vi "Coffee_machine.vi"(0 "1 Cup":bool, 1 "Water Level":dbl(slide) scale=0.0..100.0, 2 "Milk Level":dbl(slide) scale=0.0..100.0, 5 "1 Carafe":bool, 7 "Type":u32(knob) scale=0.0..2.0, 9 "Power":bool, 11 "Error In":errorcluster, 12 "Bean Level":dbl(slide) scale=0.0..100.0) -> (3 "Heating":bool, 4 "Low Water":bool, 6 "Low Bean":bool, 8 "Low Milk":bool, 10 "Purging":bool, 15 "Error Out":errorcluster)   [LabVIEW 2020]
uses:
  Typedef's/Q_Operations.ctl
  Typedef's/Data Cluster.ctl
  <vilib>/Utility/config.llb/Write Key (Boolean).vi
  <vilib>/Utility/config.llb/Read Key (Double).vi
  <vilib>/Utility/config.llb/Read Key (Boolean).vi
  <vilib>/Utility/config.llb/NI_LVConfig.lvlib
panel:
  in  "Power Shutdown?":bool
  out "Dispensing":bool
  out "Brewing":bool
  out "Grinding":bool
  out "Total Cups":dbl
  out "Elapsed Time":dbl format="%#.0f"
  out "Dispenser":dbl(slide) scale=0.0..60.0
  in  "Chamber":dbl(slide) scale=0.0..60.0
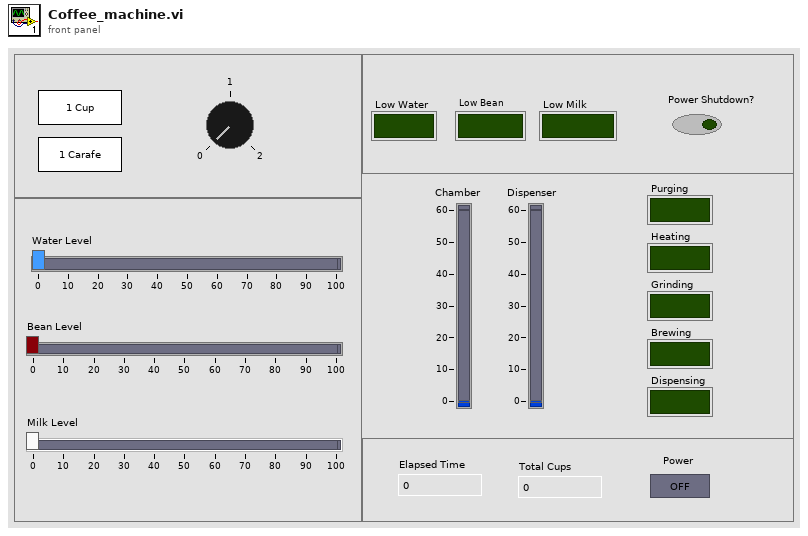
[diagram p1: front panel]
types:
  T1 = typedef "Data Cluster.ctl" = cluster{"Bean Level":dbl, "Chamber":dbl, "Dispenser":dbl, "Milk Level":dbl, "Elapsed Time":dbl, "Total Cups":dbl, "Water Level":dbl, "1 Carafe":bool, "1 Cup":bool, "Low Bean":bool, "Low Water":bool, "Low Milk":bool, "Power Shutdown?":bool, "Heating":bool, "Grinding":bool, "Brewing":bool, "Dispensing":bool, "Purging":bool, "Power":bool, "Type":u32, "Timer":cluster{"Previous Time":dbl, "Elapsed Time":dbl, "Start":bool, "Pause":bool, "Set Time":dbl}, "Sequecne":string[], "Value":dbl}
  T2 = typedef "Q_Operations.ctl" = enum16{"Create Q", "Enqueue", "Dequeue", "Enqueue N ele", "Enstack N ele", "Flush Q", "Destroy Q"}
  T3 = enum8{"Enabled", "Disabled", "Disabled and Grayed Out"}
  T4 = typedef "NI_LVConfig.lvlib/Config Data RefNum.ctl" = refnum<k1>
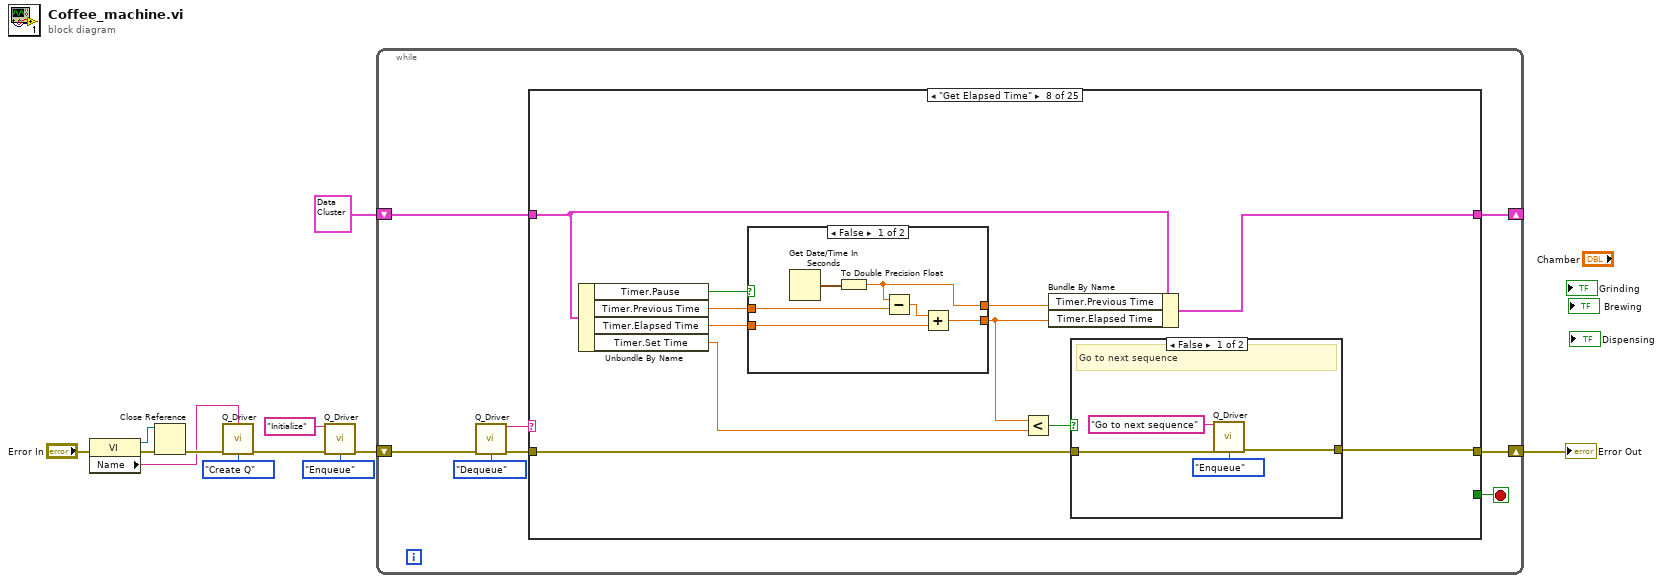
[diagram p0: block diagram]
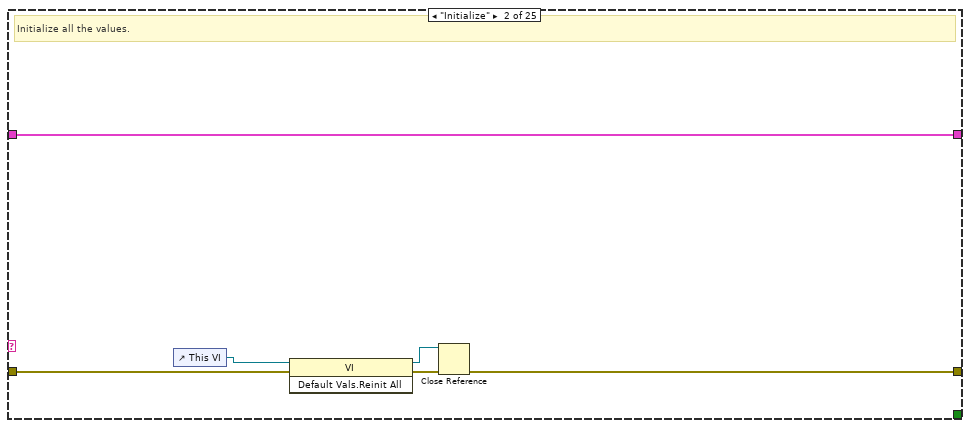
[diagram p3: hidden frame]
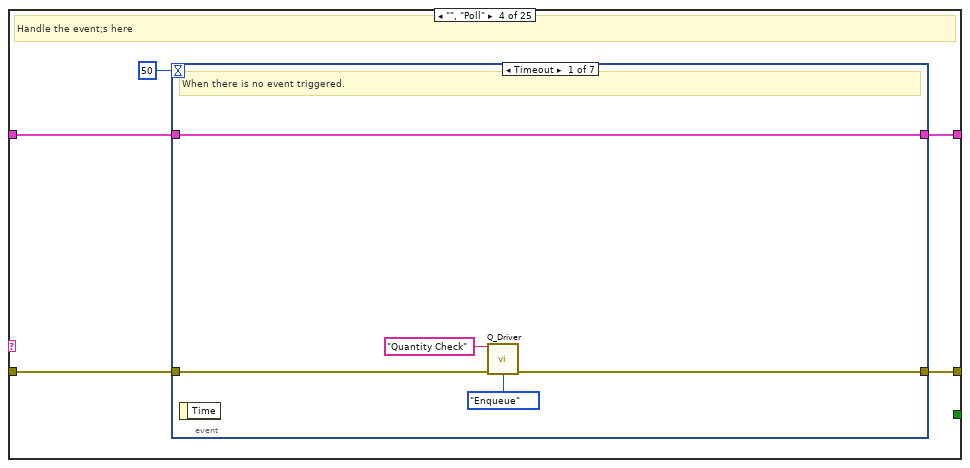
[diagram p5: hidden frame]
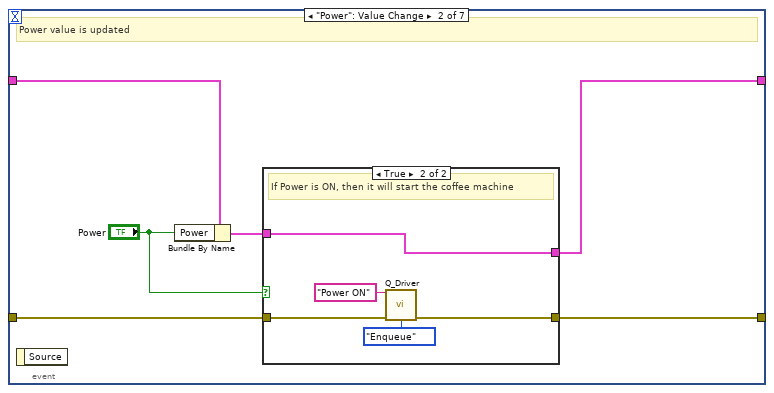
[diagram p6: hidden frame]
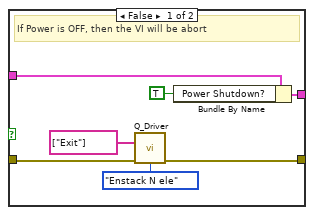
[diagram p7: hidden frame]
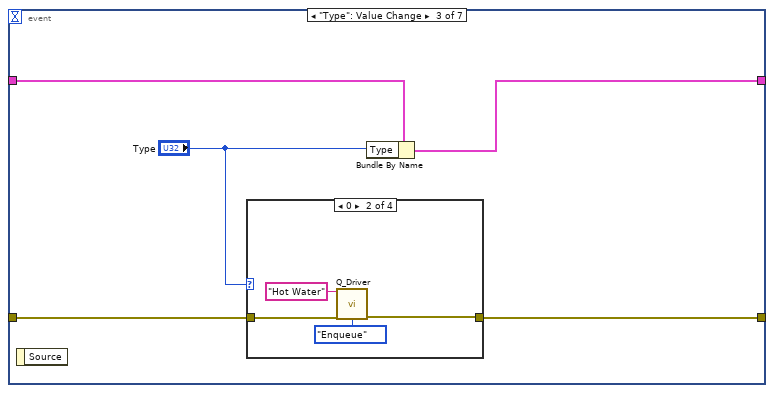
[diagram p8: hidden frame]
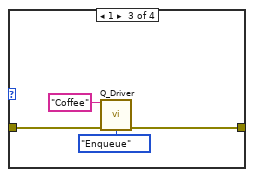
[diagram p10: hidden frame]
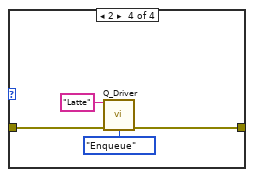
[diagram p11: hidden frame]
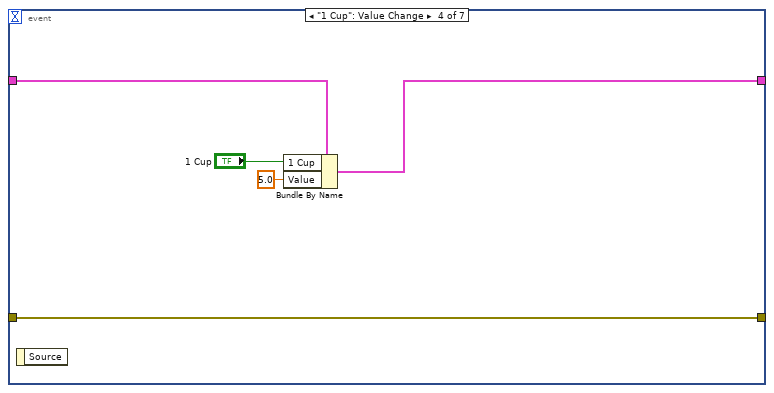
[diagram p12: hidden frame]
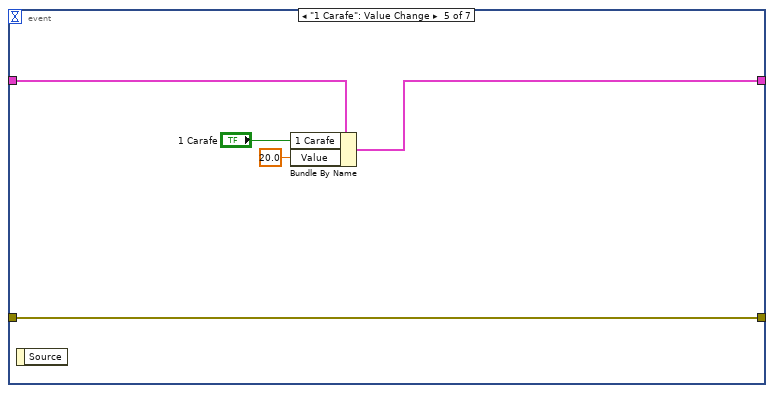
[diagram p13: hidden frame]
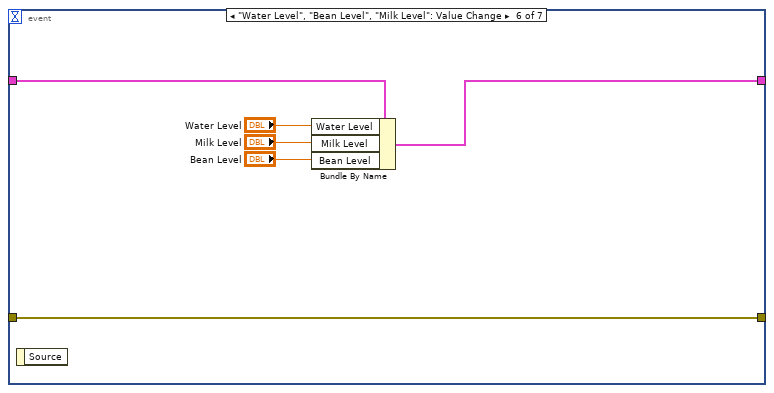
[diagram p14: hidden frame]
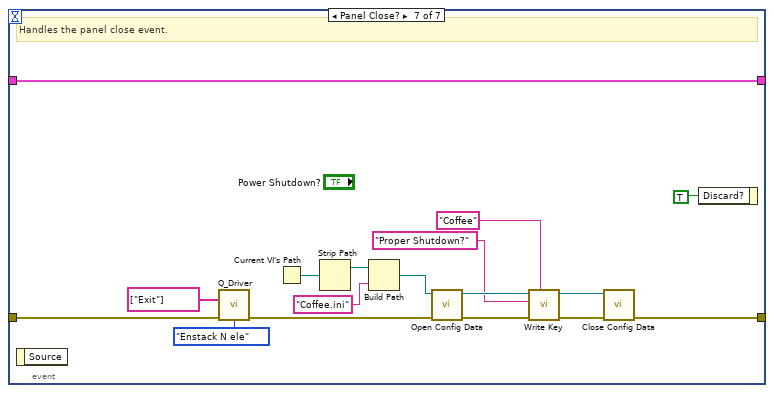
[diagram p15: hidden frame]
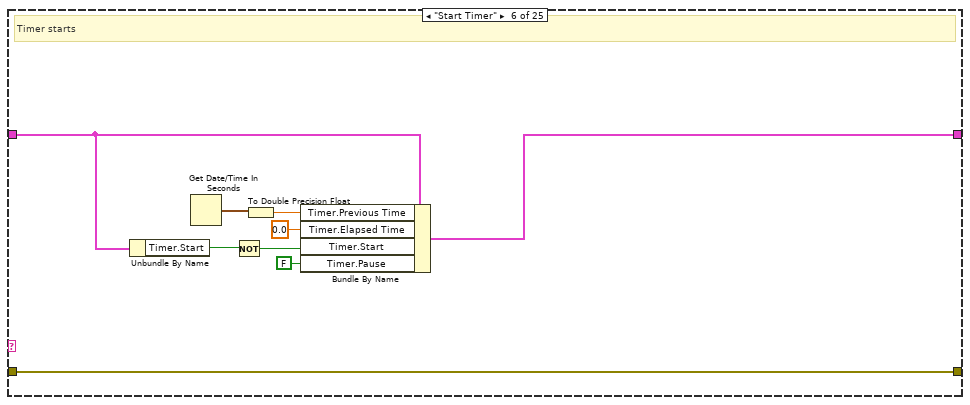
[diagram p17: hidden frame]
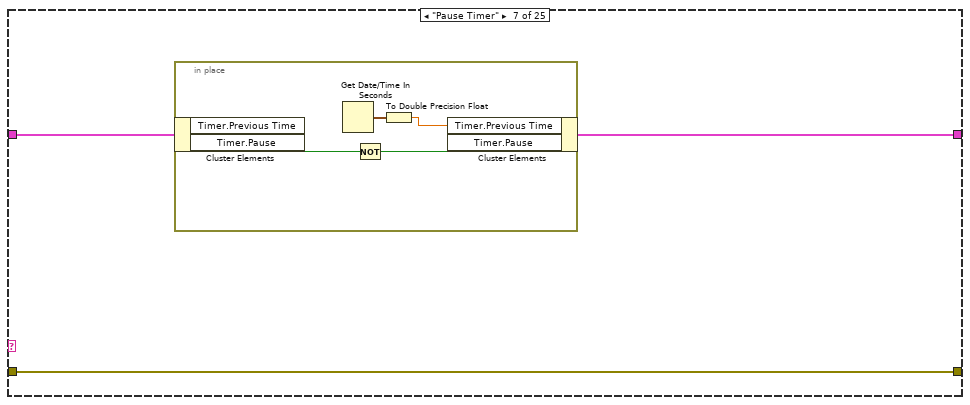
[diagram p18: hidden frame]
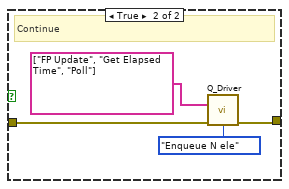
[diagram p19: hidden frame]
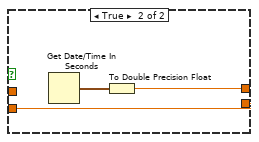
[diagram p20: hidden frame]
diagram:
  n1 = property class="VI"(error in="Error In") -> (reference out=w9:refnum<vi>, error out=w11:errorcluster, "Name"=w6:string)  [unwired: 1 in]
  n2 = Close Reference(reference=w9, error in (no error)=w11) -> (error out=w10:errorcluster)
  n3 = call "Q_Driver.vi"("Name"=w6, "Error In"=w10, "Operations"=Q_Operations."Create Q") -> ("Error Out"=w8:errorcluster)  [unwired: 11 in, 1 out]
  n4 = call "Q_Driver.vi"("State"="Initialize", "Error In"=w8, "Operations"=Q_Operations."Enqueue") -> ("Error Out"=w5:errorcluster)  [unwired: 11 in, 1 out]
  n5 = while {
    shift-right: [w16] -> w2
    shift-left: w5 -> [w19]
    shift-right: [w13] -> _
    shift-left: T1 {"Bean Level"=0.0, "Chamber"=0.0, "Dispenser"=0.0, "Milk Level"=0.0, "Elapsed Time"=0.0, "Total Cups"=0.0, "Water Level"=0.0, "1 Carafe"=FALSE, "1 Cup"=FALSE, "Low Bean"=FALSE, "Low Water"=FALSE, "Low Milk"=FALSE, "Power Shutdown?"=FALSE, "Heating"=FALSE, "Grinding"=FALSE, "Brewing"=FALSE, "Dispensing"=FALSE, "Purging"=FALSE, "Power"=FALSE, "Type"=0, "Timer"={"Previous Time"=0.0, "Elapsed Time"=0.0, "Start"=FALSE, "Pause"=FALSE, "Set Time"=0.0}, "Sequecne"=[], "Value"=0.0} -> [w14]
    stop <- w15 stop-if-true
    n6 = call "Q_Driver.vi"("Error In"=w19, "Operations"=Q_Operations."Dequeue") -> ("Dequeued Element"=w17:string, "Error Out"=w20:errorcluster)  [unwired: 12 in]
    n7 = case shown="\"Get Elapsed Time\"" w17 {
      tunnel: w20 -> [w22 w27 w30 w34 w111 w120 w123 w129 w157 w172 w181 w208 w216 w230 w241 w248 w271 w287 w289 w296 w298 w301 w307 w309 w311]
      tunnel: [w22 w23 w30 w33 w111 w120 w123 w128 w157 w164 w178 w209 w217 w237 w238 w247 w266 w287 w289 w296 w298 w302 w307 w309 w311] -> w16
      tunnel: [_ _ _ _ _ _ _ _ _ _ _ _ _ _ _ _ _ _ _ _ _ TRUE _ _ _] -> w15
      tunnel: w14 -> [w21 w24 w29 w32 w110 w118 w122 w134 w156 w165 w177 w211 w222 w233 w245 w256 w284 w286 w288 w295 w297 w304 w306 w308 w310]
      tunnel: [w21 w24 w29 w31 w110 w119 w121 w135 w156 w166 w176 w212 w223 w234 w245 w256 w285 w286 w288 w295 w297 w304 w306 w308 w310] -> w13
      frame "/**** Initialize ****/" {
      }
      frame "Initialize" {
        # "Initialize all the values."
        n8 = control-ref of="This VI"() -> (w28:refnum<vi>)
        n9 = invoke class="VI" method="Default Vals.Reinit All"(reference=w28, error in=w27) -> (reference out=w25:refnum<vi>, error out=w26:errorcluster)  [unwired: 1 in, 1 out]
        n10 = Close Reference(reference=w25, error in (no error)=w26) -> (error out=w23:errorcluster)
      }
      frame "/****Events*****/" {
      }
      frame "", "Poll" {
        # "Handle the event;s here"
        n11 = event shown="[0] Timeout" {
          selector: _ -> [_ _ _ _ _ _ _]
          dyn-events: _ -> [_ _ _ _ _ _ _]
          timeout: 50 -> [_ _ _ _ _ _ _]
          tunnel: w34 -> [w36 w44 w60 w77 w82 w87 w109]
          tunnel: [w37 w45 w59 w77 w82 w87 w93] -> w33
          tunnel: w32 -> [w40 w46 w62 w78 w86 w91 w105]
          tunnel: [w40 w41 w63 w81 w84 w92 w105] -> w31
          event Timeout {
            # "When there is no event triggered."
            n12 = event-data() -> ()  [unwired: 1 in, 1 out]
            n13 = call "Q_Driver.vi"("State"="Quantity Check", "Error In"=w36, "Operations"=Q_Operations."Enqueue") -> ("Error Out"=w37:errorcluster)  [unwired: 11 in, 1 out]
          }
          event "Power": Value Change {
            # "Power value is updated"
            n14 = event-data() -> ()  [unwired: 1 in, 1 out]
            n15 = Bundle By Name(cluster=w46, "Power"="Power") -> (w42:T1)
            n16 = case shown="True" "Power" {
              tunnel: [w52 w58] -> w45
              tunnel: w44 -> [w53 w57]
              tunnel: w42 -> [w49 w54]
              tunnel: [w48 w54] -> w41
              frame False {
                # "If Power is OFF, then the VI will be abort"
                n17 = call "Q_Driver.vi"("States[]"=string[] ["Exit"], "Error In"=w53, "Operations"=Q_Operations."Enstack N ele") -> ("Error Out"=w52:errorcluster)  [unwired: 11 in, 1 out]
                n18 = Bundle By Name(cluster=w49, "Power Shutdown?"=TRUE) -> (w48:T1)
              }
              frame True {
                # "If Power is ON, then it will start the coffee machine"
                n19 = call "Q_Driver.vi"("State"="Power ON", "Error In"=w57, "Operations"=Q_Operations."Enqueue") -> ("Error Out"=w58:errorcluster)  [unwired: 11 in, 1 out]
              }
            }
          }
          event "Type": Value Change {
            n20 = event-data() -> ()  [unwired: 1 in, 1 out]
            n21 = case shown="0" "Type" {
              tunnel: w60 -> [w64 w68 w72 w76]
              tunnel: [w64 w67 w71 w75] -> w59
              frame Default {
              }
              frame 0 {
                n22 = call "Q_Driver.vi"("State"="Hot Water", "Error In"=w68, "Operations"=Q_Operations."Enqueue") -> ("Error Out"=w67:errorcluster)  [unwired: 11 in, 1 out]
              }
              frame 1 {
                n23 = call "Q_Driver.vi"("State"="Coffee", "Error In"=w72, "Operations"=Q_Operations."Enqueue") -> ("Error Out"=w71:errorcluster)  [unwired: 11 in, 1 out]
              }
              frame 2 {
                n24 = call "Q_Driver.vi"("State"="Latte", "Error In"=w76, "Operations"=Q_Operations."Enqueue") -> ("Error Out"=w75:errorcluster)  [unwired: 11 in, 1 out]
              }
            }
            n25 = Bundle By Name(cluster=w62, "Type"="Type") -> (w63:T1)
          }
          event "1 Cup": Value Change {
            n26 = event-data() -> ()  [unwired: 1 in, 1 out]
            n27 = Bundle By Name(cluster=w78, "1 Cup"="1 Cup", "Value"=5.0 ("Cup")) -> (w81:T1)
          }
          event "1 Carafe": Value Change {
            n28 = event-data() -> ()  [unwired: 1 in, 1 out]
            n29 = Bundle By Name(cluster=w86, "1 Carafe"="1 Carafe", "Value"=20.0) -> (w84:T1)
          }
          event "Water Level", "Bean Level", "Milk Level": Value Change {
            n30 = event-data() -> ()  [unwired: 1 in, 1 out]
            n31 = Bundle By Name(cluster=w91, "Water Level"="Water Level", "Milk Level"="Milk Level", "Bean Level"="Bean Level") -> (w92:T1)
          }
          event Panel Close? {
            # "Handles the panel close event."
            n32 = event-data() -> ()  [unwired: 1 in, 1 out]
            n33 = call "Q_Driver.vi"("States[]"=string[] ["Exit"], "Error In"=w109, "Operations"=Q_Operations."Enstack N ele") -> ("Error Out"=w100:errorcluster)  [unwired: 11 in, 1 out]
            n34 = Current VI's Path() -> (path=w102:path)
            n35 = Strip Path(path=w102) -> (stripped path=w103:path)  [unwired: 1 out]
            n36 = Build Path(base path=w103, name or relative path="Coffee.ini") -> (appended path=w104:path)
            n37 = call <vilib>:"Open Config Data.vi"("error in (no error)"=w100, "configuration file path"=w104) -> ("error out"=w99:errorcluster, "refnum"=w98:T4)  [unwired: 7 in, 1 out]
            n38 = call-poly <vilib>:"Write Key.vi"("section"="Coffee", "error in (no error)"=w99, "key"="Proper Shutdown?", "refnum"=w98) -> ("error out"=w94:errorcluster, "refnum out"=w95:T4)  [unwired: 5 in, 1 out]
            n39 = call <vilib>:"Close Config Data.vi"("error in (no error)"=w94, "refnum"=w95) -> ("error out"=w93:errorcluster)  [unwired: 8 in, 1 out]
            n40 = event-data("Discard?"=TRUE) -> ()  [unwired: 1 in, 1 out]
          }
        }
      }
      frame "/****Timer Operations*****/" {
      }
      frame "Start Timer" {
        # "Timer starts"
        n41 = Unbundle By Name(w118) -> ("Timer.Start"=w117:bool)
        n42 = Get Date/Time In Seconds() -> (seconds since 1Jan1904=w115:timestamp)
        n43 = Not(x=w117) -> (.not. x?=w116:bool)
        n44 = To Double Precision Float(number=w115) -> (double precision float=w114:dbl)
        n45 = Bundle By Name(cluster=w118, "Timer.Previous Time"=w114, "Timer.Elapsed Time"=0.0, "Timer.Start"=w116, "Timer.Pause"=FALSE) -> (w119:T1)
      }
      frame "Pause Timer" {
        n46 = in-place {
          n47 = in-place-cluster #1(w122) -> ("Timer.Pause"=w127:bool)  [unwired: 1 out]
          n48 = Get Date/Time In Seconds() -> (seconds since 1Jan1904=w125:timestamp)
          n49 = Not(x=w127) -> (.not. x?=w126:bool)
          n50 = To Double Precision Float(number=w125) -> (double precision float=w124:dbl)
          n51 = in-place-cluster #1("Timer.Previous Time"=w124, "Timer.Pause"=w126) -> (w121:T1)
        }
      }
      frame "Get Elapsed Time" {
        n52 = Unbundle By Name(w134) -> ("Timer.Pause"=w138:bool, "Timer.Previous Time"=w136:dbl, "Timer.Elapsed Time"=w137:dbl, "Timer.Set Time"=w131:dbl)
        n53 = case shown="False" w138 {
          tunnel: [w147 w153] -> w133
          tunnel: w137 -> [w151 w155]
          tunnel: w136 -> [w148 _]
          tunnel: [w149 w155] -> w132
          frame False {
            n54 = Get Date/Time In Seconds() -> (seconds since 1Jan1904=w152:timestamp)
            n55 = To Double Precision Float(number=w152) -> (double precision float=w147:dbl)
            n56 = Subtract(x=w147, y=w148) -> (x-y=w150:dbl)
            n57 = Add(x=w150, y=w151) -> (x+y=w149:dbl)
          }
          frame True {
            n58 = Get Date/Time In Seconds() -> (seconds since 1Jan1904=w154:timestamp)
            n59 = To Double Precision Float(number=w154) -> (double precision float=w153:dbl)
          }
        }
        n60 = Less?(x=w132, y=w131) -> (x < y?=w130:bool)
        n61 = Bundle By Name(cluster=w134, "Timer.Previous Time"=w133, "Timer.Elapsed Time"=w132) -> (w135:T1)
        n62 = case shown="False" w130 {
          tunnel: w129 -> [w142 w145]
          tunnel: [w141 w146] -> w128
          frame False {
            # "Go to next sequence"
            n63 = call "Q_Driver.vi"("State"="Go to next sequence", "Error In"=w142, "Operations"=Q_Operations."Enqueue") -> ("Error Out"=w141:errorcluster)  [unwired: 11 in, 1 out]
          }
          frame True {
            # "Continue"
            n64 = call "Q_Driver.vi"("States[]"=string[] ["FP Update", "Get Elapsed Time", "Poll"], "Error In"=w145, "Operations"=Q_Operations."Enqueue N ele") -> ("Error Out"=w146:errorcluster)  [unwired: 11 in, 1 out]
          }
        }
      }
      frame "/****Functionality****/" {
      }
      frame "Power ON" {
        n65 = Current VI's Path() -> (path=w175:path)
        n66 = Strip Path(path=w175) -> (stripped path=w174:path)  [unwired: 1 out]
        n67 = Build Path(base path=w174, name or relative path="Coffee.ini") -> (appended path=w171:path)
        n68 = call <vilib>:"Open Config Data.vi"("error in (no error)"=w172, "configuration file path"=w171) -> ("error out"=w169:errorcluster, "refnum"=w170:T4)  [unwired: 7 in, 1 out]
        n69 = call-poly <vilib>:"Read Key.vi"("section"="Coffee", "error in (no error)"=w169, "key"="Total Cups", "refnum"=w170) -> ("error out"=w161:errorcluster, "value"=w162:dbl, "refnum out"=w159:T4)  [unwired: 4 in, 1 out]
        n70 = call <vilib>:"Close Config Data.vi"("error in (no error)"=w161, "refnum"=w159) -> ("error out"=w160:errorcluster)  [unwired: 8 in, 1 out]
        n71 = Bundle By Name(cluster=w165, "Total Cups"=w162) -> (w166:T1)
        n72 = call "Q_Driver.vi"("States[]"=string[] ["FP Update", "Power Update"], "Error In"=w160, "Operations"=Q_Operations."Enqueue N ele") -> ("Error Out"=w164:errorcluster)  [unwired: 11 in, 1 out]
      }
      frame "Power Update" {
        # "Power status sequence is updated"
        n73 = Current VI's Path() -> (path=w185:path)
        n74 = Strip Path(path=w185) -> (stripped path=w186:path)  [unwired: 1 out]
        n75 = Build Path(base path=w186, name or relative path="Coffee.ini") -> (appended path=w187:path)
        n76 = call <vilib>:"Open Config Data.vi"("error in (no error)"=w181, "configuration file path"=w187) -> ("error out"=w189:errorcluster, "refnum"=w188:T4)  [unwired: 7 in, 1 out]
        n77 = call-poly <vilib>:"Read Key.vi"("section"="Coffee", "error in (no error)"=w189, "key"="Proper Shutdown?", "refnum"=w188) -> ("error out"=w179:errorcluster, "value"=w180:bool)  [unwired: 4 in, 2 out]
        n78 = case shown="False" w180 {
          tunnel: w179 -> [w195 w201]
          tunnel: [w196 w200] -> w178
          tunnel: w177 -> [w192 w197]
          tunnel: [w191 w197] -> w176
          frame False {
            # "If the VI is aborted , then Purging process starts"
            n79 = call "Q_Driver.vi"("States[]"=string[] ["Start Timer", "Purging", ""], "Error In"=w195, "Operations"=Q_Operations."Enqueue N ele") -> ("Error Out"=w196:errorcluster)  [unwired: 11 in, 1 out]
            n80 = Bundle By Name(cluster=w192, "Sequecne"=string[] ["Purging", "Heating"]) -> (w191:T1)
          }
          frame True {
            # "If Power is OFF, then Heating process starts"
            n81 = call "Q_Driver.vi"("States[]"=string[] ["Start Timer", "Heating"], "Error In"=w201, "Operations"=Q_Operations."Enqueue N ele") -> ("Error Out"=w200:errorcluster)  [unwired: 11 in, 1 out]
          }
        }
      }
      frame "Heating" {
        n82 = call "Q_Driver.vi"("State"="Get Elapsed Time" ("States[]"), "Error In"=w208, "Operations"=Q_Operations."Enqueue") -> ("Error Out"=w209:errorcluster)  [unwired: 11 in, 1 out]
        n83 = Bundle By Name(cluster=w211, "Purging"=FALSE, "Heating"=TRUE, "Chamber"=0.0, "Dispenser"=0.0, "Timer.Set Time"=5.0) -> (w212:T1)
      }
      frame "Purging" {
        n84 = call "Q_Driver.vi"("State"="Get Elapsed Time", "Error In"=w216, "Operations"=Q_Operations."Enqueue") -> ("Error Out"=w217:errorcluster)  [unwired: 11 in, 1 out]
        n85 = Bundle By Name(cluster=w222, "Heating"=FALSE, "Purging"=TRUE, "Chamber"=0.0, "Dispenser"=0.0, "Timer.Set Time"=4.0) -> (w223:T1)
      }
      frame "Go to next sequence" {
        n86 = Unbundle By Name(w233) -> ("Sequecne"=w231:string[])
        n87 = Delete From Array(array=w231, index=0) -> (array with subset deleted=w229:string[])  [unwired: 1 in, 1 out]
        n88 = Index Array(array=w229, index=0) -> (element=w225:string)
        n89 = Empty String/Path?(string/path=w225) -> (empty?=w227:bool)
        n90 = Select(t="Default state", s=w227, f=w225) -> (s? t:f=w224:string)
        n91 = Bundle By Name(cluster=w233, "Sequecne"=w229, "Timer.Elapsed Time"=0.0) -> (w234:T1)
        n92 = call "Q_Driver.vi"("State"=w224, "Error In"=w230, "Operations"=Q_Operations."Enqueue") -> ("Error Out"=w237:errorcluster)  [unwired: 11 in, 1 out]
      }
      frame "Default state" {
        n93 = control-ref of="This VI"() -> (w242:refnum<vi>)
        n94 = invoke class="VI" method="Default Vals.Reinit All"(reference=w242, error in=w241) -> (reference out=w244:refnum<vi>, error out=w243:errorcluster)  [unwired: 1 in, 1 out]
        n95 = Close Reference(reference=w244, error in (no error)=w243) -> (error out=w239:errorcluster)
        n96 = property on="Power" class="Bool (strict)"(error in=w239, "Value"=TRUE ("Power")) -> (error out=w238:errorcluster)  [unwired: 1 in, 1 out]
      }
      frame "Quantity Check" {
        w252 = 30.0 ("y")
        n97 = Unbundle By Name(w256) -> ("Water Level"=w255:dbl, "Bean Level"=w254:dbl, "Milk Level"=w253:dbl)
        n98 = Greater?(x=w255, y=w252) -> (0:w246:bool)
        n99 = Greater?(x=w254, y=w252) -> (0:w251:bool)
        n100 = Greater?(x=w253, y=w252) -> (0:w250:bool)
        n101 = Compound Arithmetic op=OR(w246, w251, w250) -> (w249:bool)
        n102 = case shown="False" w249 {
          tunnel: w248 -> [w258 w260]
          tunnel: [w257 w261] -> w247
          frame False {
            n103 = property on="Type" class="Knob (strict)"(error in=w258, "DisabledEnum"=T3."Disabled and Grayed Out" ("Disabled")) -> (error out=w257:errorcluster)  [unwired: 1 in, 1 out]
          }
          frame True {
            n104 = property on="Type" class="Knob (strict)"(error in=w260, "DisabledEnum"=T3."Enabled" ("Disabled")) -> (error out=w261:errorcluster)  [unwired: 1 in, 1 out]
          }
        }
      }
      frame "Hot Water" {
        n105 = Unbundle By Name(w284) -> ("Dispenser"=w283:dbl, "Value"=w277:dbl, "Water Level"=w281:dbl, "Total Cups"=w275:dbl)
        n106 = Add(x=w275, y=4.0) -> (x+y=w273:dbl)
        n107 = Increment(x=w275) -> (x+1=w276:dbl)
        n108 = Equal?(x=w277, y=5.0) -> (x = y?=w278:bool)
        n109 = Add(x=w283, y=w277) -> (x+y=w282:dbl)
        n110 = Subtract(x=w281, y=w277) -> (x-y=w280:dbl)
        n111 = Select(t=w276, s=w278, f=w273) -> (s? t:f=w272:dbl)
        n112 = Bundle By Name(cluster=w284, "Dispensing"=TRUE, "Dispenser"=w282, "Water Level"=w280, "Total Cups"=w272, "Timer.Set Time"=5.0, "Timer.Elapsed Time"=0.0) -> (w285:T1)
        n113 = call "Q_Driver.vi"("States[]"=string[] ["Get Elapsed Time"], "Error In"=w271, "Operations"=Q_Operations."Enqueue N ele") -> ("Error Out"=w267:errorcluster)  [unwired: 11 in, 1 out]
        n114 = property on="Water Level" class="Slide (strict)"(error in=w267, "Indicator"=TRUE) -> (error out=w266:errorcluster)  [unwired: 1 in, 1 out]
      }
      frame "Coffee" {
      }
      frame "Latte" {
      }
      frame "FP Update" {
        n115 = Unbundle By Name(w295) -> ("Total Cups"=→"Total Cups":dbl, "Timer.Elapsed Time"=→"Elapsed Time":dbl, "Heating"=→"Heating":bool, "Purging"=→"Purging":bool, "Dispenser"=→"Dispenser":dbl)
      }
      frame "/***** Exit******/" {
      }
      frame "Exit" {
        # "Handles the exit state"
        n116 = call "Q_Driver.vi"("Error In"=w301, "Operations"=Q_Operations."Flush Q") -> ("Error Out"=w303:errorcluster)  [unwired: 12 in, 1 out]
        n117 = call "Q_Driver.vi"("Error In"=w303, "Operations"=Q_Operations."Destroy Q") -> ("Error Out"=w302:errorcluster)  [unwired: 12 in, 1 out]
      }
      frame "/**** Error States ****/" {
      }
      frame "Error" {
        # "When there is error occured."
      }
      frame "Developer Error", Default {
        # "When there is any developer mistakes"
      }
    }
  }
  "Error Out" <- w2
